vi "cbc radio label fixup.vi"(8 "error in (no error)":errorcluster) -> (0 "error out":errorcluster, 3 "New string":string, 11 "Response":string)   [LabVIEW 2013]
panel:
  out "ZPL":string
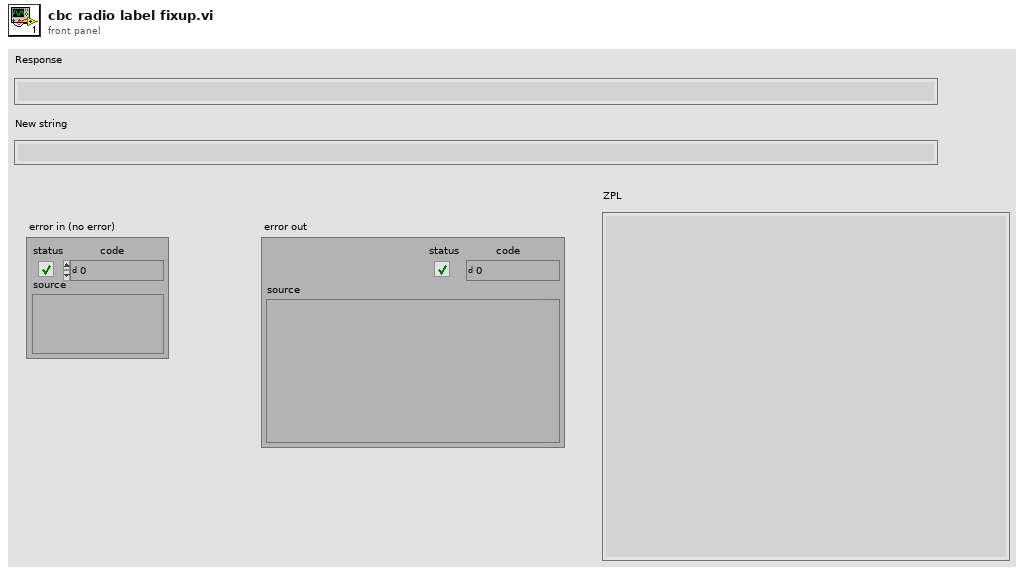
[diagram p1: front panel]
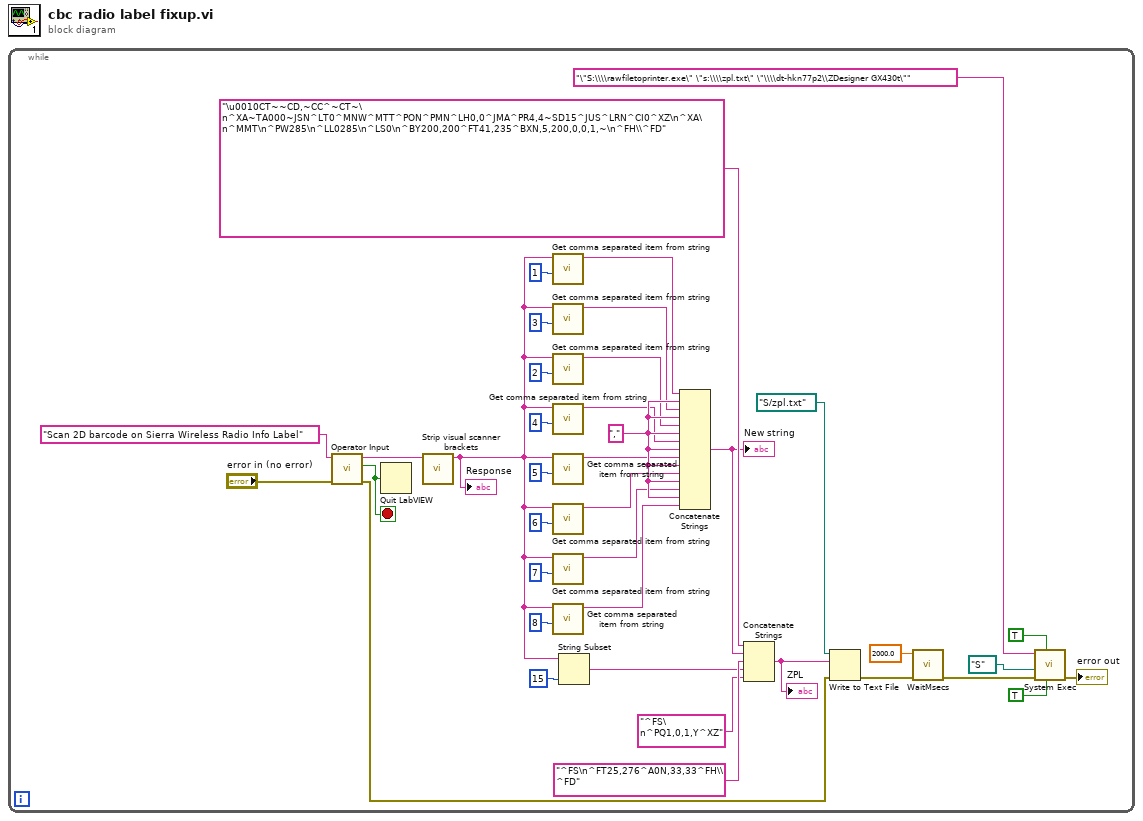
[diagram p0: block diagram]
diagram:
  n1 = while {
    stop <- w6 stop-if-true
    w28 = "," ("string")
    n2 = call "Operator Input.vi"("error in (no error)"="error in (no error)", "Message"="Scan 2D barcode on Sierra Wireless Radio Info Label") -> ("error out"=w8:errorcluster, "Stop button hit"=w6:bool, "Response"=w20:string)  [unwired: 7 in]
    n3 = Quit LabVIEW(quit? (T)=w6) -> ()
    n4 = call "Strip visual scanner brackets.vi"("Work order scan"=w20) -> ("result string"=w4:string)  [unwired: 9 in, 1 out]
    "Response" <- w4
    n5 = call "Get comma separated item from string.vi"("Field Num (1-n)"=u32 1, "String to parse with commas"=w4) -> ("Item string value"=w29:string)  [unwired: 8 in, 1 out]
    n6 = call "Get comma separated item from string.vi"("Field Num (1-n)"=u32 3, "String to parse with commas"=w4) -> ("Item string value"=w27:string)  [unwired: 8 in, 1 out]
    n7 = call "Get comma separated item from string.vi"("Field Num (1-n)"=u32 2, "String to parse with commas"=w4) -> ("Item string value"=w26:string)  [unwired: 8 in, 1 out]
    n8 = call "Get comma separated item from string.vi"("Field Num (1-n)"=u32 4, "String to parse with commas"=w4) -> ("Item string value"=w25:string)  [unwired: 8 in, 1 out]
    n9 = call "Get comma separated item from string.vi"("Field Num (1-n)"=u32 5, "String to parse with commas"=w4) -> ("Item string value"=w24:string)  [unwired: 8 in, 1 out]
    n10 = call "Get comma separated item from string.vi"("Field Num (1-n)"=u32 6, "String to parse with commas"=w4) -> ("Item string value"=w23:string)  [unwired: 8 in, 1 out]
    n11 = call "Get comma separated item from string.vi"("Field Num (1-n)"=u32 7, "String to parse with commas"=w4) -> ("Item string value"=w22:string)  [unwired: 8 in, 1 out]
    n12 = call "Get comma separated item from string.vi"("Field Num (1-n)"=u32 8, "String to parse with commas"=w4) -> ("Item string value"=w21:string)  [unwired: 8 in, 1 out]
    n13 = String Subset(string=w4, length (rest)=15 ("length (rest)")) -> (substring=w2:string)  [unwired: 1 in]
    n14 = Concatenate Strings(w29, w28, w27, w28, w26, w28, w25, w28, w24, w28, w23, w28, w22, w28, w21) -> (w18:string)
    "New string" <- w18
    n15 = Concatenate Strings("\u0010CT~~CD,~CC^~CT~\n^XA~TA000~JSN^LT0^MNW^MTT^PON^PMN^LH0,0^JMA^PR4,4~SD15^JUS^LRN^CI0^XZ\n^XA\n^MMT\n^PW285\n^LL0285\n^LS0\n^BY200,200^FT41,235^BXN,5,200,0,0,1,~\n^FH\\^FD", w18, "^FS\n^FT25,276^A0N,33,33^FH\\^FD", w2, "^FS\n^PQ1,0,1,Y^XZ") -> (w12:string)
    "ZPL" <- w12
    n16 = Write to Text File(file (use dialog)=path "S:/zpl.txt", text=w12, error in=w8) -> (error out=w13:errorcluster)  [unwired: 1 in, 2 out]
    n17 = call "WaitMsecs.vi"("error in (no error)"=w13, "Wait Msecs"=2000.0) -> ("error out"=w15:errorcluster)  [unwired: 9 in]
    n18 = call <vilib>:"System Exec.vi"("run minimized? (F)"=TRUE, "wait until completion? (T)"=TRUE, "error in (no error)"=w15, "working directory"=path "S:/", "command line"="\"S:\\\\rawfiletoprinter.exe\" \"s:\\\\zpl.txt\" \"\\\\dt-hkn77p2\\ZDesigner GX430t\"" ("string")) -> ("error out"=→"error out":errorcluster)  [unwired: 3 in, 3 out]
  }
